vi "GV N pixel clock per line.vi"() -> ()   [LabVIEW 2017]
panel:
  out "N pixel clock per line":i16
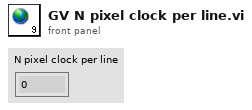
[diagram p1: front panel]
diagram:
